vi "Zero Phase Filter (obs).vi"   [LabVIEW 2018, in "NI_AALBase.lvlib"]
doc: "Applies a zero phase filter to an input sequence <B>X</B>. Wire data to the <B>X</B> input to determine the polymorphic instance to use or manually select the instance."
uses:
  NI_AALBase.lvlib
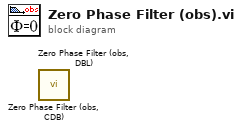
[diagram p0: block diagram]
diagram:
  n1 = call "Zero Phase Filter (obs, CDB).vi"() -> ()  [unwired: 10 in, 2 out]
  n2 = call "Zero Phase Filter (obs, DBL).vi"() -> ()  [unwired: 10 in, 2 out]
